vi "Generate Event.vi"(8 "error in (no error)":errorcluster, 9 "Data":variant, 10 "Event Type":T1=enum."Button 0 Click", 11 "Sender":string) -> (0 "error out":errorcluster)   [LabVIEW 2019, in "GaitDAQ UI Event.lvlib"]
uses:
  GaitDAQ UI Event.lvlib
  Event Type.ctl
  <userlib>/JUL/Event Message Module/Event Message Library/Event Action.ctl
panel:
  # "Input"
  # "Output"
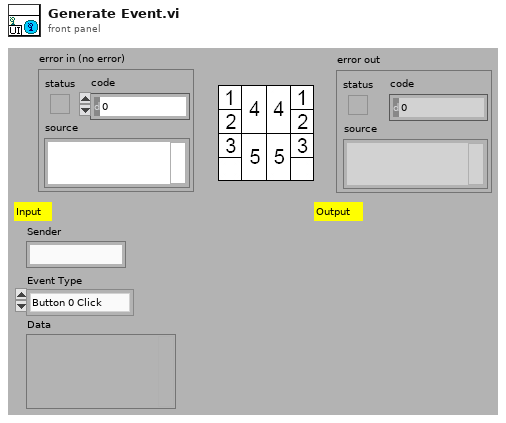
[diagram p1: front panel]
types:
  T1 = typedef "GaitDAQ UI Event.lvlib/Event Type.ctl" = enum16{"Default", "Initialize Finish", "Button 0 Click", "Panel Close", "Exit"}
  T2 = typedef "Event Action.ctl" = enum16{"Default", "Generate Event", "Register", "Unregister(Customize Event and Register)", "Unregister(All Events In Customize Register)", "Unregister(All Registers In Customize Event)", "Get Register Table"}
  T3 = cluster{"Event Type":T1, "Sender":string, "Data":variant}
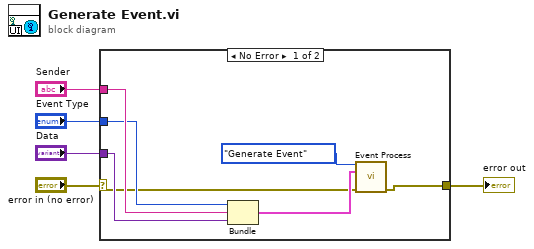
[diagram p0: block diagram]
diagram:
  n1 = case shown="No Error" "error in (no error)" {
    selector: "error in (no error)" -> [w7 w13]
    tunnel: [w6 w13] -> w2
    tunnel: "Event Type" -> [w9 _]
    tunnel: "Data" -> [w10 _]
    tunnel: "Sender" -> [w11 _]
    frame No Error {
      n2 = Bundle("Event Type"=w9, "Sender"=w11, "Data"=w10) -> (w8:T3)  [unwired: 1 in]
      n3 = call "Event Process.vi"("Event Action"=Event_Action."Generate Event", "Generate Event Data"=w8, "error in (no error)"=w7) -> ("error out"=w6:errorcluster)  [unwired: 11 in, 1 out]
    }
    frame Error {
    }
  }
  "error out" <- w2
